vi "store_last_RowData.vi"() -> ()   [LabVIEW 2019]
uses:
  RowData_Type.ctl
panel:
  in  "RowData":T1
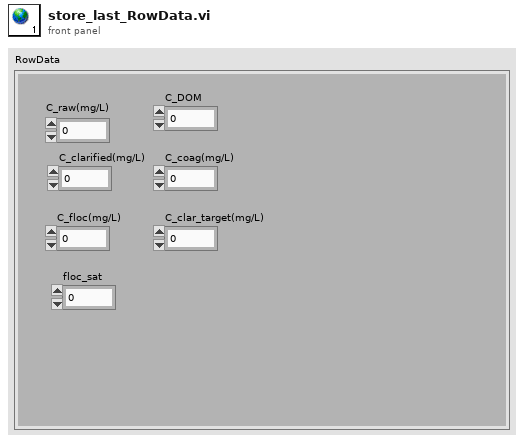
[diagram p1: front panel]
types:
  T1 = typedef "RowData_Type.ctl" = cluster{"C_raw(mg/L)":dbl, "C_clarified(mg/L)":dbl, "C_floc(mg/L)":dbl, "floc_sat":dbl, "C_DOM":dbl, "C_coag(mg/L)":dbl, "C_clar_target(mg/L)":dbl}
diagram:
